vi "ModifyAttribute1.vi"(0 "reference in":refnum<class "G#SubClass1.lvclass">, 1 "Lock time (ms)":u32, 5 "error in (no error)":errorcluster, 7 "status":bool) -> (14 "reference out":refnum<class "G#SubClass1.lvclass">, 19 "error out":errorcluster)   [LabVIEW 2010, in "G#SubClass1.lvclass"]
uses:
  G#SubClass1.lvclass
  G#BaseClass1_class/G#BaseClass1.lvclass
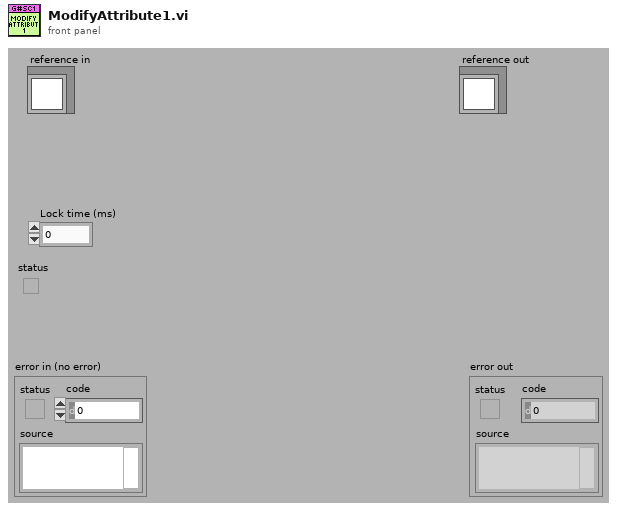
[diagram p1: front panel]
types:
  T1 = typedef "G#BaseClass1.lvclass/ObjectAttributesRef.ctl" = refnum<data-value>
  T2 = typedef "G#SubClass1.lvclass/ObjectAttributesRef.ctl" = refnum<data-value>
  T3 = typedef "G#SubClass1.lvclass/ObjectAttributes.ctl" = cluster{"SubNumeric":dbl, "TestQueue":refnum<queue>}
  T4 = typedef "G#BaseClass1.lvclass/ObjectAttributes.ctl" = cluster{"Numeric":dbl, "Array":dbl[]}
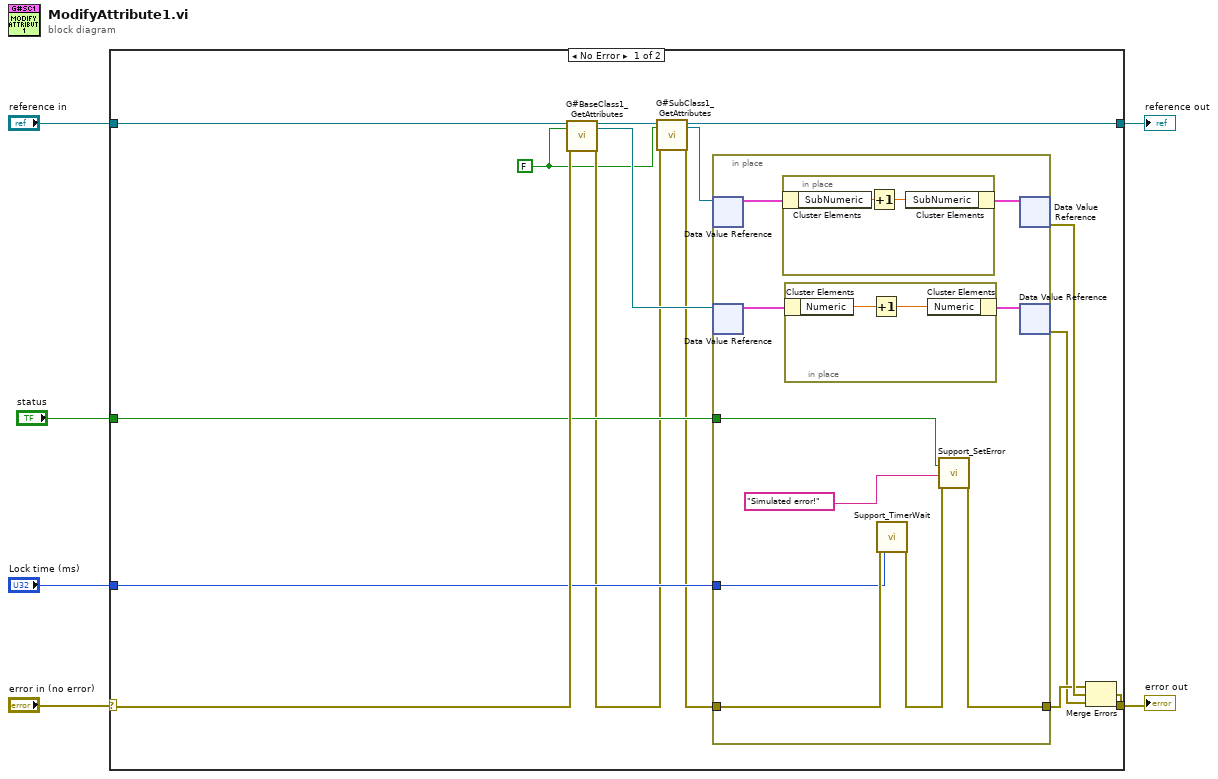
[diagram p0: block diagram]
diagram:
  n1 = case shown="No Error" "error in (no error)" {
    selector: "error in (no error)" -> [w17 w37]
    tunnel: [w21 w37] -> w5
    tunnel: [w11 w36] -> w3
    tunnel: "reference in" -> [w18 w36]
    tunnel: "Lock time (ms)" -> [w14 _]
    tunnel: "status" -> [w13 _]
    frame No Error {
      w8 = FALSE ("return data")
      n2 = call "G#BaseClass1_GetAttributes.vi"("reference in"=w18, "return data? (T)"=w8, "error in (no error)"=w17) -> ("reference out"=w12:refnum<class "G#SubClass1.lvclass">, "attributes ref"=w16:T1, "error out"=w10:errorcluster)  [unwired: 13 in, 1 out]
      n3 = call "G#SubClass1_GetAttributes.vi"("reference in"=w12, "return data? (T)"=w8, "error in (no error)"=w10) -> ("reference out"=w11:refnum<class "G#SubClass1.lvclass">, "attributes ref"=w7:T2, "error out"=w9:errorcluster)  [unwired: 13 in, 1 out]
      n4 = in-place {
        in-place-border: w9 -> [w27]
        in-place-border: [w24] -> w19
        in-place-border: w14 -> [w26]
        in-place-border: w13 -> [w22]
        n5 = in-place-dvr #1(w7) -> (w30:T3)  [unwired: 1 out]
        n6 = in-place-dvr #2(w16) -> (w29:T4)  [unwired: 1 out]
        n7 = in-place {
          n8 = in-place-cluster #3(w30) -> ("SubNumeric"=w35:dbl)
          n9 = Increment(x=w35) -> (x+1=w34:dbl)
          n10 = in-place-cluster #3("SubNumeric"=w34) -> (w31:T3)
        }
        n11 = in-place {
          n12 = in-place-cluster #4(w29) -> ("Numeric"=w33:dbl)
          n13 = Increment(x=w33) -> (x+1=w32:dbl)
          n14 = in-place-cluster #4("Numeric"=w32) -> (w28:T4)
        }
        n15 = call "Support_TimerWait.vi"("error in (no error)"=w27, "milliseconds to wait"=w26) -> ("error out"=w25:errorcluster)  [unwired: 17 in]
        n16 = call "Support_SetError.vi"("status"=w22, "source"="Simulated error!", "error in (no error)"=w25) -> ("error out"=w24:errorcluster)  [unwired: 16 in]
        n17 = in-place-dvr #1(w31) -> (w20:errorcluster)  [unwired: 1 out]
        n18 = in-place-dvr #2(w28) -> (w15:errorcluster)  [unwired: 1 out]
      }
      n19 = Merge Errors(w19, w20, w15) -> (w21:errorcluster)
    }
    frame Error {
    }
  }
  "error out" <- w5
  "reference out" <- w3
